vi "showFrontEnd.vi"(8 "error in (no error)":errorcluster, 11 "CameraControlViewer in":refnum<class "CameraControlViewer.lvclass">) -> (0 "error out":errorcluster, 3 "CameraControlViewer out":refnum<class "CameraControlViewer.lvclass">)   [LabVIEW 2011, in "Views.lvlib" / "Camera.lvlib" / "CameraControlViewer.lvclass"]
uses:
  CameraControlViewer.lvclass
  CameraControlViewer.lvclass/CameraControlViewer.ctl
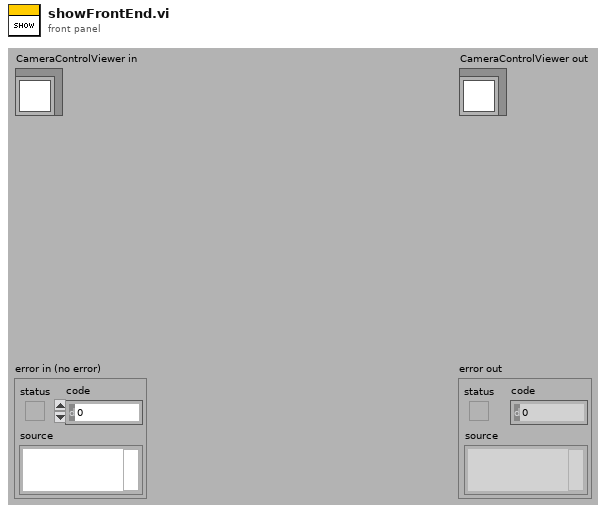
[diagram p1: front panel]
types:
  T1 = enum32{"Invalid", "Standard", "Closed", "Hidden", "Minimized", "Maximized"}
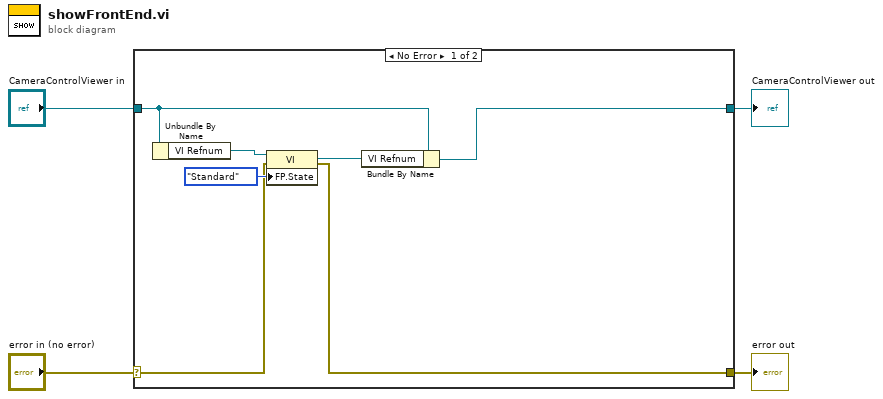
[diagram p0: block diagram]
diagram:
  n1 = case shown="No Error" "error in (no error)" {
    selector: "error in (no error)" -> [w9 w13]
    tunnel: [w8 w13] -> w3
    tunnel: [w5 w12] -> w1
    tunnel: "CameraControlViewer in" -> [w6 w12]
    frame No Error {
      n2 = Unbundle By Name(w6) -> ("VI Refnum"=w11:refnum<vi>)
      n3 = property class="VI"(reference=w11, error in=w9, "FP.State"=T1."Standard" ("Front Panel Window:State")) -> (reference out=w7:refnum<vi>, error out=w8:errorcluster)
      n4 = Bundle By Name(cluster=w6, "VI Refnum"=w7) -> (w5:refnum<class "CameraControlViewer.lvclass">)
    }
    frame Error {
    }
  }
  "error out" <- w3
  "CameraControlViewer out" <- w1
